vi "Update User[ ].vi"(8 "error in (no error)":errorcluster, 10 "Message":variant, 11 "Telegram Class in":refnum<class "Telegram Class.lvclass">) -> (0 "error out":errorcluster, 3 "Telegram Class out":refnum<class "Telegram Class.lvclass">)   [LabVIEW 2015, in "Telegram Library.lvlib" / "Telegram Class.lvclass"]
doc: "Created IvanLis by LabVIEW Portal\nProfile: http://labviewportal.org/memberlist.php?mode=viewprofile&u=987\neMail: IvanLisanov@gMail.com\nTelegram: https://t.me/IvanLis"
uses:
  Telegram Class.lvclass
  JSON Library/TypeDef/User.ctl
  TypeDef/User.ctl
  Telegram Class.lvclass/Telegram Class.ctl
  JSON Library/JSON Library.lvlib
  Telegram Library.lvlib
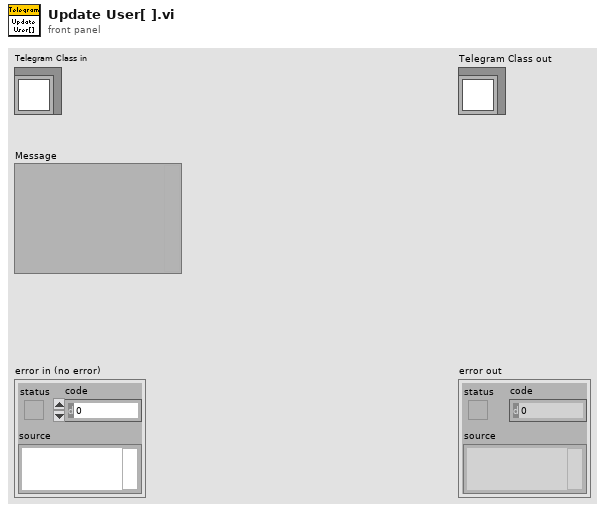
[diagram p1: front panel]
types:
  T1 = typedef "JSON Library.lvlib/user.ctl" = cluster{"@type":string, "id":i64, "first_name":string, "last_name":string, "username":string, "phone_number":string}
  T2 = typedef "Telegram Library.lvlib/User.ctl" = cluster{"id":i64, "phone_number":string, "username":string, "last_name":string, "first_name":string}
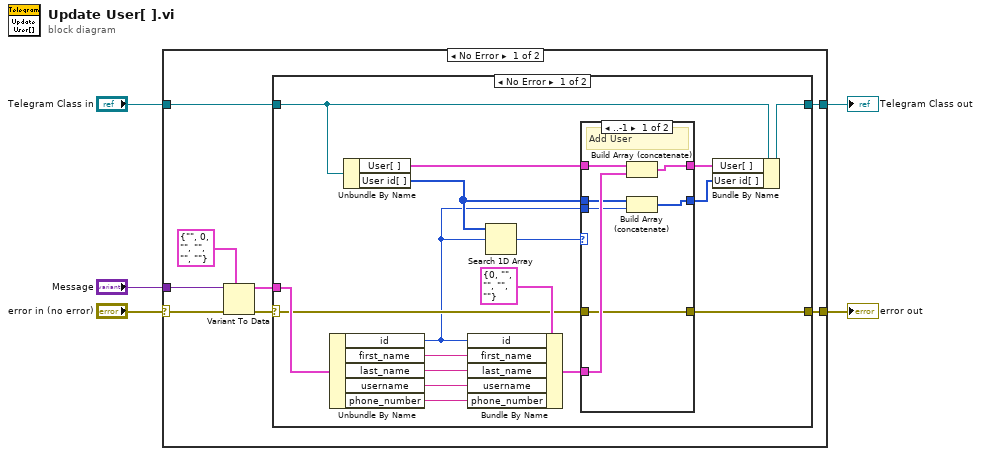
[diagram p0: block diagram]
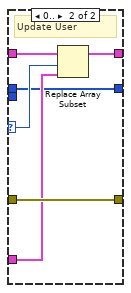
[diagram p2: hidden frame]
diagram:
  n1 = case shown="No Error" "error in (no error)" {
    selector: "error in (no error)" -> [w13 w47]
    tunnel: [w8 w47] -> w4
    tunnel: [w6 w46] -> w2
    tunnel: "Telegram Class in" -> [w7 w46]
    tunnel: "Message" -> [w11 _]
    frame No Error {
      n2 = Variant To Data(error in=w13, type=T1 {"@type"="", "id"=0, "first_name"="", "last_name"="", "username"="", "phone_number"=""} ("user"), Variant=w11) -> (data=w10:T1, error out=w9:errorcluster)
      n3 = case shown="No Error" w9 {
        selector: w9 -> [w21 w45]
        tunnel: w10 -> [w30 _]
        tunnel: [w24 w45] -> w8
        tunnel: w7 -> [w18 w44]
        tunnel: [w17 w44] -> w6
        frame No Error {
          n4 = Unbundle By Name(w30) -> ("id"=w15:i64, "first_name"=w29:string, "last_name"=w28:string, "username"=w25:string, "phone_number"=w27:string)
          n5 = Unbundle By Name(w18) -> ("User[ ]"=w20:T2[], "User id[ ]"=w16:i64[])
          n6 = Bundle By Name(cluster=T2 {"id"=0, "phone_number"="", "username"="", "last_name"="", "first_name"=""} ("User"), "id"=w15, "first_name"=w29, "last_name"=w28, "username"=w25, "phone_number"=w27) -> (w26:T2)
          n7 = Search 1D Array(1D array=w16, element=w15) -> (index of element=w22:i32)  [unwired: 1 in]
          n8 = case shown="..-1" w22 {
            selector: w22 -> [_ w40]
            tunnel: w21 -> [w35 w43]
            tunnel: w26 -> [w36 w41]
            tunnel: [w35 w43] -> w24
            tunnel: w20 -> [w37 w42]
            tunnel: [w34 w39] -> w19
            tunnel: w16 -> [w33 w38]
            tunnel: w15 -> [w32 _]
            tunnel: [w31 w38] -> w14
            frame ..-1 {
              # "Add User"
              n9 = Build Array (concatenate)(w37, w36) -> (w34:T2[])
              n10 = Build Array (concatenate)(w33, w32) -> (w31:i64[])
            }
            frame 0.. {
              # "Update User"
              n11 = Replace Array Subset(array=w42, new element=w41, index=w40) -> (w39:T2[])
            }
          }
          n12 = Bundle By Name(cluster=w18, "User[ ]"=w19, "User id[ ]"=w14) -> (w17:refnum<class "Telegram Class.lvclass">)
        }
        frame Error {
        }
      }
    }
    frame Error {
    }
  }
  "error out" <- w4
  "Telegram Class out" <- w2
